vi "String to Boolean.vi"(11 "booleanString":string) -> (3 "state":bool)   [LabVIEW 2012]
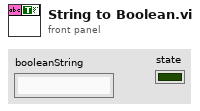
[diagram p1: front panel]
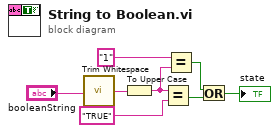
[diagram p0: block diagram]
diagram:
  n1 = call <vilib>:"Trim Whitespace.vi"("string"="booleanString") -> ("trimmed string"=w7:string)  [unwired: 1 in]
  n2 = To Upper Case(1:w7) -> (0:w5:string)
  n3 = Equal?(x=w5, y="TRUE") -> (x = y?=w2:bool)
  n4 = Equal?(x="1", y=w5) -> (x = y?=w3:bool)
  n5 = Or(x=w3, y=w2) -> (x .or. y?=→"state":bool)
